vi "ObtainMessageQue.vi"(8 "error in":errorcluster, 9 "max queue size (-1, unlimited)":i32=-1, 10 "Name":string) -> (0 "error out":errorcluster, 1 "created new?":bool, 2 "Name out":string, 3 "message que out":T1)   [LabVIEW 2018, in "MessageQue.lvlib"]
doc: "Create a queue with the Message data type.\n\nBolder Software LLC"
uses:
  MessageQue.lvlib
  MessageQue.ctl
  MessageCluster.ctl
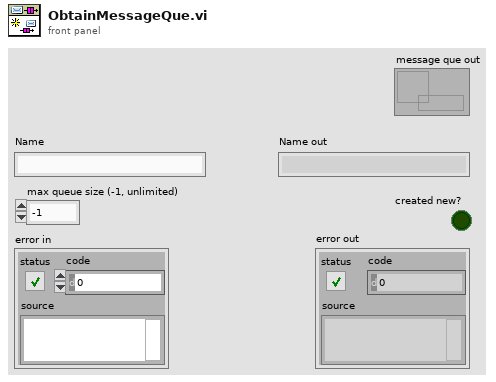
[diagram p1: front panel]
types:
  T1 = typedef "MessageQue.lvlib/MessageQue.ctl" = refnum<queue>
  T2 = typedef "MessageQue.lvlib/MessageCluster.ctl" = cluster{"Command":string, "Payload":variant}
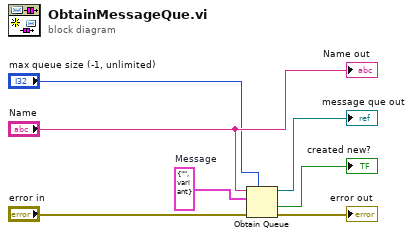
[diagram p0: block diagram]
diagram:
  w7 = T2 {"Command"="", "Payload"=variant}  # Message
  n1 = Obtain Queue(max queue size (-1, unlimited)="max queue size (-1, unlimited)", name (unnamed)="Name", element data type=w7, error in (no error)="error in") -> (queue out=→"message que out":refnum<queue>, created new?=→"created new?":bool, error out=→"error out":errorcluster)  [unwired: 1 in]
  "Name out" <- "Name"
